vi "ReadReportedError.vi"(6 "timeout in ms (-1)":i32=-1, 8 "error in":errorcluster, 11 "error processor in":refnum<class "ErrorProcessor.lvclass">) -> (0 "error out":errorcluster, 1 "error received?":bool, 2 "error message":T1, 3 "error processor out":refnum<class "ErrorProcessor.lvclass">, 4 "terminate loop?":bool)   [LabVIEW 2013, in "CLM_ErrorHandler.lvlib" / "ErrorProcessor.lvclass"]
uses:
  ErrorProcessor.lvclass
  ErrorMessage.ctl
  ErrorProcessor.lvclass/ErrorProcessor.ctl
  <vilib>/CLM/LocalMessenger/PriorityLocalMessage/CLM_PriorityLocalMessage.lvclass/CLM_PriorityLocalMessage.ctl
  <vilib>/CLM/LocalMessenger/LocalMessage_Queue/CLM_LocalMessage_Queue.lvclass/CLM_LocalMessage_Queue.ctl
  <vilib>/CLM/LocalMessenger/PriorityLocalMessage/ReadMessageCluster.vi
  <vilib>/CLM/LocalMessenger/LocalMessage_Queue/DestroyQueueMessage.vi
  <vilib>/CLM/LocalMessenger/LocalMessage_Queue/ReadQueueMessage_Cluster.vi
  <vilib>/CLM/LocalMessenger/PriorityLocalMessage/BufferIndexToPriority.vi
  <vilib>/CLM/LocalMessenger/PriorityLocalMessage/FG_NamedQueues.vi
  <vilib>/CLM/LocalMessenger/PriorityLocalMessage/CLM_PriorityLocalMessage.lvclass
  CLM_ErrorHandler.lvlib
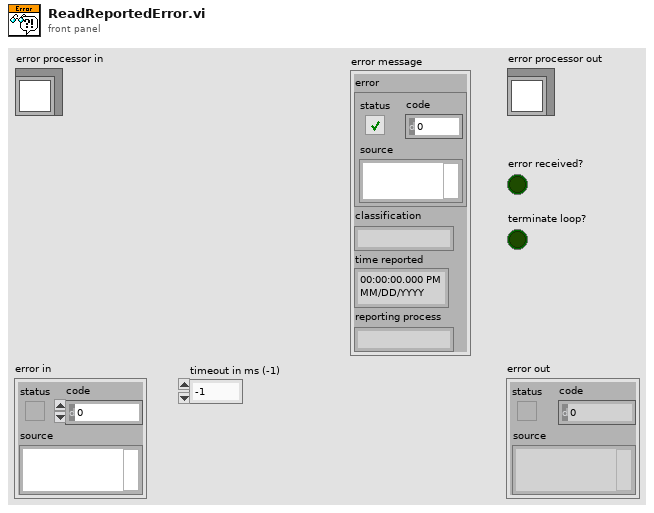
[diagram p1: front panel]
types:
  T1 = typedef "CLM_ErrorHandler.lvlib/ErrorMessage.ctl" = cluster{"error":errorcluster, "classification":string, "time reported":timestamp, "reporting process":string}
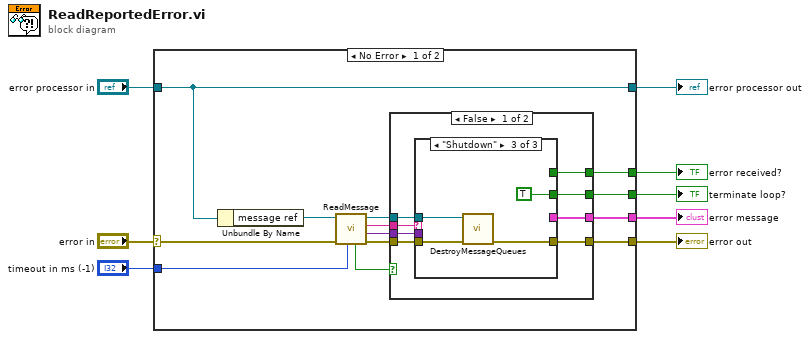
[diagram p0: block diagram]
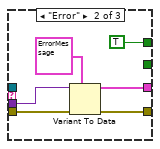
[diagram p3: hidden frame]
diagram:
  n1 = case shown="No Error" "error in" {
    selector: "error in" -> [w19 w43]
    tunnel: [w13 w43] -> w7
    tunnel: [w21 w42] -> w5
    tunnel: "error processor in" -> [w21 w42]
    tunnel: "timeout in ms (-1)" -> [w18 _]
    tunnel: [w12 _] -> w3
    tunnel: [w11 _] -> w2
    tunnel: [w9 _] -> w1
    frame No Error {
      n2 = Unbundle By Name(w21) -> ("message ref"=w20:refnum<class "CLM_PriorityLocalMessage.lvclass">)
      n3 = call <vilib>:"ReadMessage.vi"("timeout in ms (-1)"=w18, "error in"=w19, "message ref in"=w20) -> ("error out"=w14:errorcluster, "data"=w15:variant, "name"=w16:string, "message ref out"=w10:refnum<class "CLM_PriorityLocalMessage.lvclass">, "timed out?"=w17:bool)  [unwired: 2 in, 2 out]
      n4 = case shown="False" w17 {
        tunnel: w16 -> [w29 _]
        tunnel: w15 -> [w28 _]
        tunnel: w14 -> [w27 w41]
        tunnel: [w25 w41] -> w13
        tunnel: [w26 _] -> w12
        tunnel: [w24 _] -> w11
        tunnel: w10 -> [w23 _]
        tunnel: [w22 _] -> w9
        frame False {
          n5 = case shown="\"Shutdown\"" w29 {
            tunnel: w28 -> [_ w35 _]
            tunnel: w27 -> [w30 w36 w38]
            tunnel: [_ w33 _] -> w26
            tunnel: [w30 w32 w37] -> w25
            tunnel: [_ TRUE _] -> w24
            tunnel: w23 -> [_ _ w39]
            tunnel: [_ _ TRUE] -> w22
            frame Default {
            }
            frame "Error" {
              n6 = Variant To Data(error in=w36, type=T1 {"error"={"status"=FALSE, "code"=0, "source"=""}, "classification"="", "time reported"=timestamp(0 s since 1904-01-01), "reporting process"=""} ("error message"), Variant=w35) -> (data=w33:T1, error out=w32:errorcluster)
            }
            frame "Shutdown" {
              n7 = call <vilib>:"DestroyMessageQueues.vi"("error in"=w38, "message ref in"=w39) -> ("error out"=w37:errorcluster)  [unwired: 8 in, 1 out]
            }
          }
        }
        frame True {
        }
      }
    }
    frame Error {
    }
  }
  "error out" <- w7
  "error processor out" <- w5
  "error message" <- w3
  "terminate loop?" <- w1
  "error received?" <- w2
